vi "Scan String.vi"(9 "Class Number":i32=3, 10 "String":string, 11 "Numeric in":i32) -> (3 "Numeric out":i32)   [LabVIEW 2017]
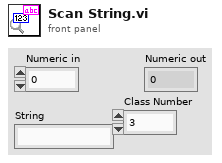
[diagram p1: front panel]
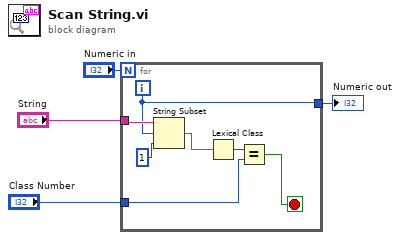
[diagram p0: block diagram]
diagram:
  n1 = for {
    N: "Numeric in" -> [_]
    tunnel: "String" -> [w10]
    tunnel: [w7] -> w2
    tunnel: "Class Number" -> [w5]
    i -> [w7]
    stop <- w6 stop-if-true
    n2 = String Subset(string=w10, offset (0)=w7, length (rest)=1 ("length (rest)")) -> (substring=w8:string)
    n3 = Lexical Class(1:w8) -> (0:w11:i16)
    n4 = Equal?(x=w11, y=w5) -> (x = y?=w6:bool)
  }
  "Numeric out" <- w2
